vi "Intra-Move Items.vi"(4 "indent":i32, 6 "Insertion index":i32, 8 "error in (no error)":errorcluster, 9 "Copy?":bool, 10 "Indices to move":i32[](array[numeric]), 11 "BetterBoxHandle in":refnum<class "BetterBoxHandle.lvclass">) -> (0 "error out":errorcluster, 3 "BetterBoxHandle out":refnum<class "BetterBoxHandle.lvclass">)   [LabVIEW 2020, in "BetterDragAndDrop.lvlib" / "BetterBoxHandle.lvclass"]
uses:
  BetterBoxHandle.lvclass
  C:/DSCE code/Open-source/betterdraganddrop_GIT/Source/Classes/BetterHandle/BetterHandle.lvclass
  BetterHandle/BetterHandle.lvclass/BetterHandle.ctl
  17a33ecd-a91c-412f-a565-520f4c39e11a.vi
  BetterHandle/BetterHandle.lvclass
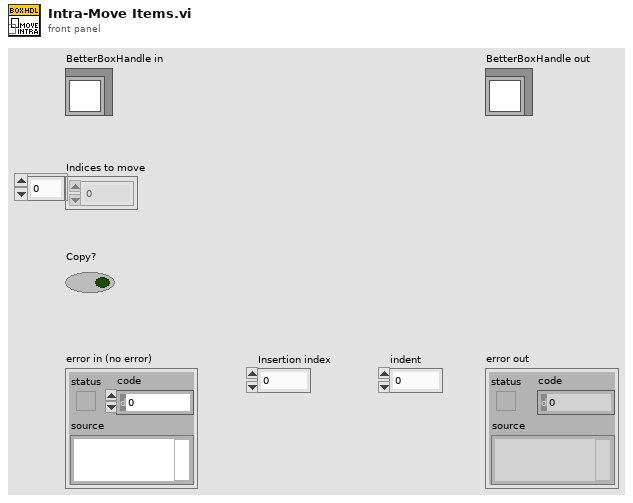
[diagram p1: front panel]
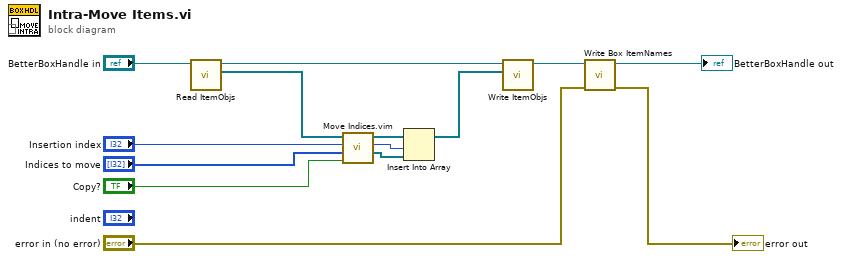
[diagram p0: block diagram]
diagram:
  n1 = call "Read ItemObjs.vi"("BetterHandle in"="BetterBoxHandle in") -> ("ItemObjs"=w14:refnum<class "BetterItem.lvclass">[], "BetterHandle out"=w13:refnum<class "BetterBoxHandle.lvclass">)  [unwired: 9 in]
  n2 = call "Move Indices.vim"("Copy?"="Copy?", "Indices to move"="Indices to move", "insertion index"="Insertion index", "Array"=w14) -> ("elements to be inserted"=w2:refnum<class "BetterItem.lvclass">[], "new insertion index"=w3:i32, "modified array"=w4:refnum<class "BetterItem.lvclass">[])  [unwired: 5 in]
  n3 = Insert Into Array(array=w4, index=w3, new element=w2) -> (w1:refnum<class "BetterItem.lvclass">[])
  n4 = call "Write ItemObjs.vi"("ItemObjs"=w1, "BetterHandle in"=w13) -> ("BetterHandle out"=w12:refnum<class "BetterBoxHandle.lvclass">)  [unwired: 9 in]
  n5 = call-dynamic "Write Box ItemNames.vi"("error in (no error)"="error in (no error)", "BetterBoxHandle in"=w12) -> ("error out"=→"error out":errorcluster, "BetterBoxHandle out"=→"BetterBoxHandle out":refnum<class "BetterBoxHandle.lvclass">)  [unwired: 8 in]
